vi "SavePMC2.vi"(0 "PMC path":path, 1 "Filename":string, 2 "instrument file path":path, 3 "Pass/Fail":string, 4 "Operator ID":string, 5 "error in":errorcluster, 6 "Serial no.":string, 8 "Datetime":string) -> (19 "error out":errorcluster)   [LabVIEW 2024, in "Test_2.lvlib"]
uses:
  Test_2.lvlib
  Launcher/Launcher_DTU.lvlib
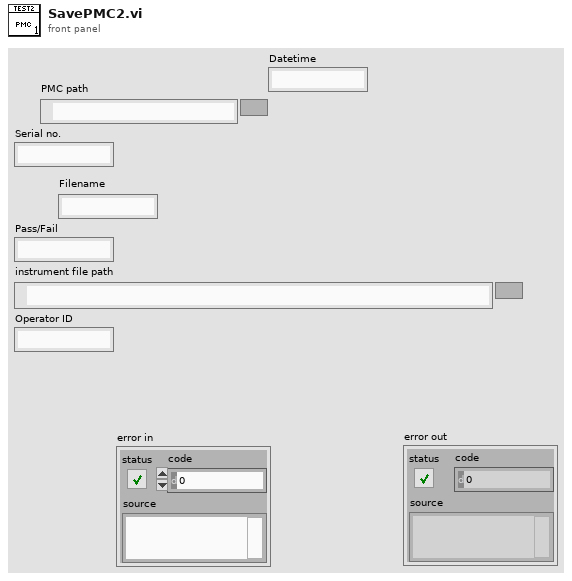
[diagram p1: front panel]
types:
  T1 = enum16{"Read", "Write", "All_sections", "All_values", "Remove key&section"}
  T2 = enum16{"open", "replace", "create", "open or create", "replace or create", "replace or create with confirmation"}
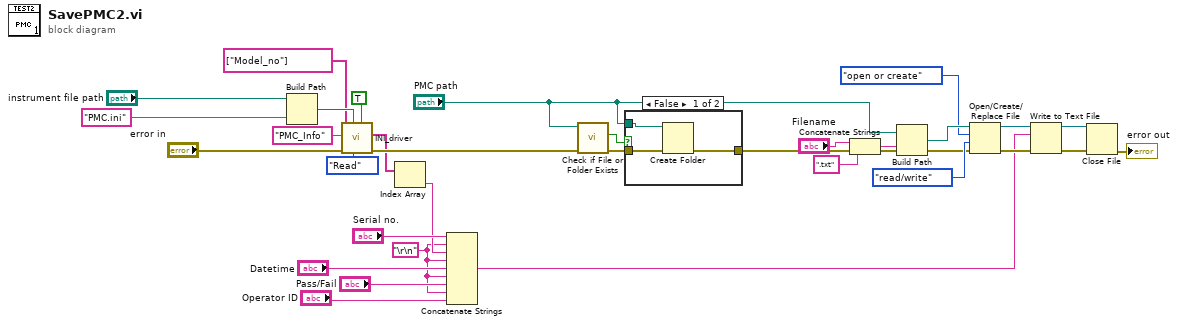
[diagram p0: block diagram]
diagram:
  w11 = "\r\n"
  n1 = Build Path(base path="instrument file path", name or relative path="PMC.ini") -> (appended path=w21:path)
  n2 = call "INI_driver.vi"("create file if necessary (T)"=TRUE, "Enum"=T1."Read", "instrument file path"=w21, "error in (no error)"="error in", "Section"="PMC_Info", "Key_name"=string[] ["Model_no"]) -> ("error out"=w24:errorcluster, "Values out"=w15:string[])  [unwired: 2 in, 2 out]
  n3 = Index Array(array=w15) -> (element=w14:string)  [unwired: 1 in]
  n4 = Concatenate Strings("Serial no.", w11, w14, w11, "Datetime", w11, "Pass/Fail", w11, "Operator ID") -> (w8:string)
  n5 = call <vilib>:"Check if File or Folder Exists.vi"("error in (no error)"=w24, "path"="PMC path") -> ("error out"=w4:errorcluster, "file or folder exists?"=w1:bool)  [unwired: 7 in, 1 out]
  n6 = case shown="False" w1 {
    tunnel: w4 -> [w35 w36]
    tunnel: [w34 w36] -> w3
    tunnel: "PMC path" -> [w33 _]
    frame False {
      n7 = Create Folder(path (use dialog)=w33, error in=w35) -> (error out=w34:errorcluster)  [unwired: 1 in, 2 out]
    }
    frame True {
    }
  }
  n8 = Concatenate Strings("Filename", ".txt" ("string")) -> (w30:string)
  n9 = Build Path(base path="PMC path", name or relative path=w30) -> (appended path=w29:path)
  n10 = Open/Create/Replace File(file path (use dialog)=w29, error in=w3, operation (0:open)=T2."open or create", access (0:read/write)=enum16{"read/write", "read-only", "write-only"}."read/write") -> (refnum out=w25:refnum<file>, error out=w26:errorcluster)  [unwired: 2 in, 1 out]
  n11 = Write to Text File(file (use dialog)=w25, text=w8, error in=w26) -> (refnum out=w6:refnum<file>, error out=w7:errorcluster)  [unwired: 1 in, 1 out]
  n12 = Close File(refnum=w6, error in=w7) -> (error out=→"error out":errorcluster)  [unwired: 1 out]
